vi "readRS232.vi"(8 "error in (no error)":errorcluster, 11 "FPGA in":refnum<class "FPGA.lvclass">) -> (0 "error out":errorcluster, 2 "Data":u8[](array[numeric]), 3 "FPGA out":refnum<class "FPGA.lvclass">)   [LabVIEW 2016, in "FPGA.lvclass"]
uses:
  FPGA.lvclass
  FPGA.lvclass/FPGA.ctl
  <vilib>/Utility/error.llb/Error Cluster From Error Code.vi
  <vilib>/rvi/errors/niLvFpgaAdjustHostInterfaceError.vi
  <vilib>/rvi/interface/nirviMethod/nirviMethod.xnode
  <vilib>/FPGAPlugInAG/Dynamic/niLvFpga_ReadFifo_Dynamic.vi
  <vilib>/rvi/errors/niLvFpgaMergeErrorWithErrorCode.vi
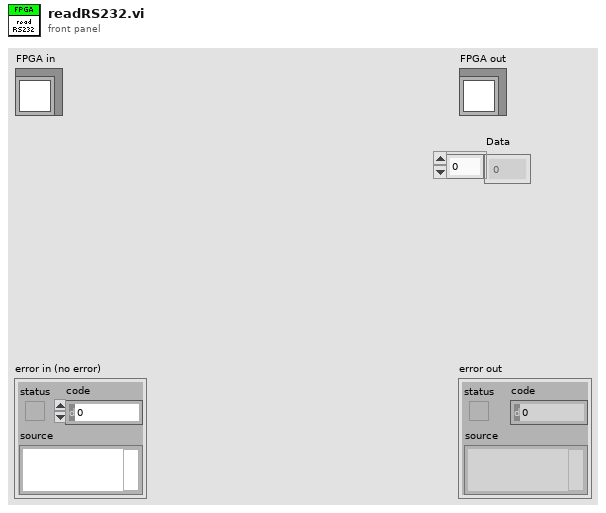
[diagram p1: front panel]
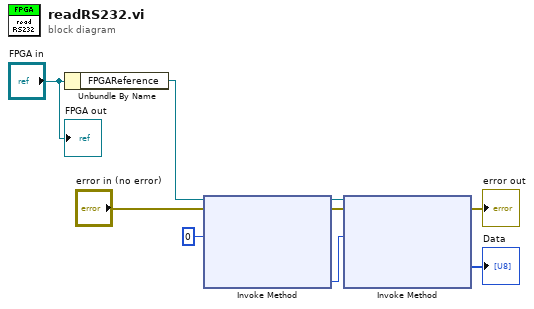
[diagram p0: block diagram]
diagram:
  n1 = Unbundle By Name("FPGA in") -> ("FPGAReference"=w8:refnum<k20>)
  n2 = xnode "Invoke Method"("FPGA VI Reference In"=w8, "error in"="error in (no error)", "Number of Elements"=u32 0) -> ("FPGA VI Reference Out"=w7:refnum<k20>, "error out"=w6:errorcluster, "Elements Remaining"=w3:u32)  [unwired: 1 in, 1 out]
  n3 = xnode "Invoke Method"("FPGA VI Reference In"=w7, "error in"=w6, "Number of Elements"=w3) -> ("error out"=→"error out":errorcluster, "Data"=→"Data":u8[])  [unwired: 1 in, 2 out]
  "FPGA out" <- "FPGA in"
